vi "输入数据.vi"(4 "数据输入界限:最小值":dbl, 6 "数据输入界限:最大值":dbl, 7 "前面板窗口:标题":string="输入数据", 8 "错误输入（无错误）":errorcluster, 10 "默认值":dbl, 11 "提示":string) -> (0 "错误输出":errorcluster, 3 "输入数据":dbl format="%#_8g")   [LabVIEW 2020]
panel:
  in  "确定":bool
  out "字符串":string
  in  "输入":dbl format="%#_8g"
  in  "启用":bool=TRUE
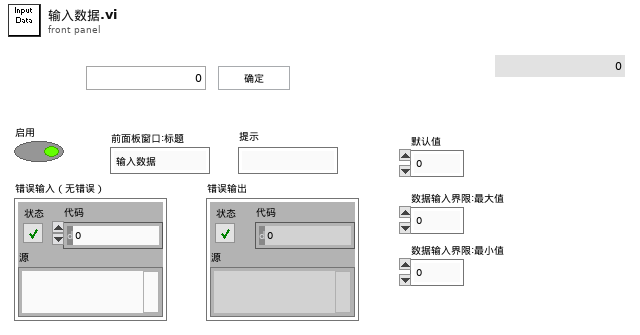
[diagram p1: front panel]
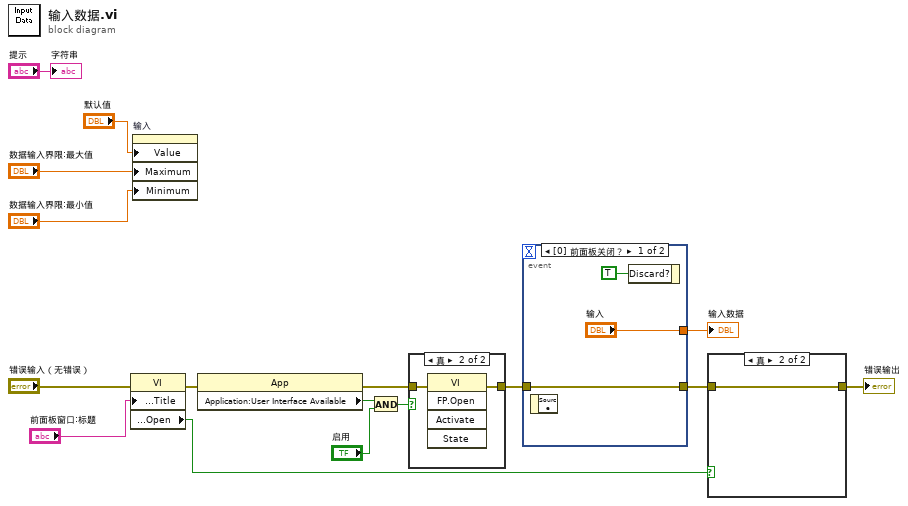
[diagram p0: block diagram]
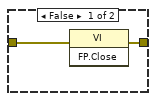
[diagram p2: hidden frame]
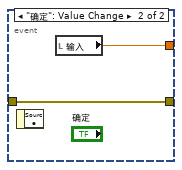
[diagram p4: hidden frame]
diagram:
  n1 = property class="VI"(error in="错误输入（无错误）", "Front Panel.Title"="前面板窗口:标题") -> (error out=w7:errorcluster, "Front Panel Window:Open"=w10:bool)  [unwired: 1 in, 1 out]
  n2 = property on="输入" class="DigNum (严格)"("Value"="默认值", "Maximum"="数据输入界限:最大值", "Minimum"="数据输入界限:最小值") -> ()  [unwired: 2 in, 2 out]
  n3 = property class="App"(error in=w7) -> (error out=w6:errorcluster, "Application:User Interface Available"=w4:bool)  [unwired: 1 in, 1 out]
  n4 = And(x=w4, y="启用") -> (x .and. y?=w14:bool)
  n5 = case shown="真" w14 {
    tunnel: w6 -> [w17 w19]
    tunnel: [w17 w18] -> w13
    frame False {
    }
    frame True {
      n6 = invoke class="VI" method="FP.Open"(error in=w19) -> (error out=w18:errorcluster)  [unwired: 4 in, 4 out]
    }
  }
  n7 = event shown="[0] 前面板关闭？" {
    selector: _ -> [_ _]
    dyn-events: _ -> [_ _]
    timeout: _ -> [_ _]
    tunnel: ["输入" w24] -> w16
    tunnel: w13 -> [w21 w23]
    tunnel: [w21 w23] -> w15
    event Panel Close? {
      n8 = event-data() -> ()  [unwired: 1 in, 1 out]
      n9 = event-data("Discard?"=TRUE ("放弃？")) -> ()  [unwired: 1 in, 1 out]
    }
    event "确定": Value Change {
      n10 = event-data() -> ()  [unwired: 1 in, 1 out]
      n11 = local read "输入"() -> (w24:dbl)
    }
  }
  "输入数据" <- w16
  n12 = case shown="真" w10 {
    tunnel: w15 -> [w26 w27]
    tunnel: [w25 w27] -> w11
    frame False {
      n13 = invoke class="VI" method="FP.Close"(error in=w26) -> (error out=w25:errorcluster)  [unwired: 2 in, 2 out]
    }
    frame True {
    }
  }
  "错误输出" <- w11
  "字符串" <- "提示"
